vi "Find the extremal value using 2nd polynomial.vi"(5 "Y":dbl[](array[numeric]), 6 "X":dbl[](array[numeric])) -> (0 "Best Polynomial Fit":dbl[](array[numeric]), 1 "Polynomial Coefficients":dbl[](array[numeric]), 2 "Xm":dbl)   [LabVIEW 2014]
uses:
  <vilib>/Analysis/6fits.llb/General Linear Fit Algorithm.ctl
  <vilib>/Analysis/NI_AALPro.lvlib
panel:
  out "XY Graph":cluster{"X":dbl[], "Y":dbl[]}[](graph)
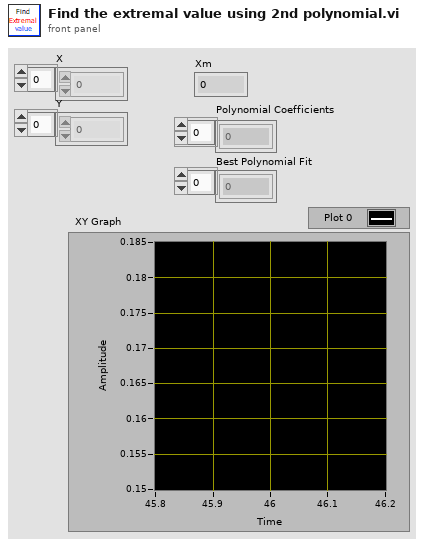
[diagram p1: front panel]
types:
  T1 = typedef "NI_AALPro.lvlib/General Linear Fit Algorithm.ctl" = u16
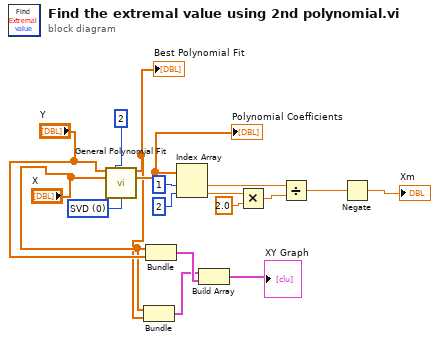
[diagram p0: block diagram]
diagram:
  w7 = T1 0 items=["SVD", "Givens", "Givens2", "Householder", "LU Decomposition", "Cholesky", "SVD for Rank Deficient H"] ("algorithm")
  n1 = call <vilib>:"General Polynomial Fit.vi"("Y"="Y", "polynomial order"=2, "X"="X", "algorithm"=w7) -> ("Best Polynomial Fit"=w4:dbl[], "Polynomial Coefficients"=w9:dbl[])  [unwired: 8 in, 2 out]
  "Best Polynomial Fit" <- w4
  "Polynomial Coefficients" <- w9
  n2 = Bundle("X"="X", "Best Polynomial Fit"=w4) -> (w2:cluster{"X":dbl[], "Best Polynomial Fit":dbl[]})  [unwired: 1 in]
  n3 = Bundle("X"="X", "Y"="Y") -> (w3:cluster{"X":dbl[], "Y":dbl[]})  [unwired: 1 in]
  n4 = Index Array(array=w9, index #1=1 ("index"), index #2=2 ("index")) -> (element #1=w14:dbl, element #2=w12:dbl)
  n5 = Build Array(w2, w3) -> (→"XY Graph":cluster{"X":dbl[], "Y":dbl[]}[])
  n6 = Multiply(x=w12, y=2.0) -> (x*y=w15:dbl)
  n7 = Divide(x=w14, y=w15) -> (x/y=w16:dbl)
  n8 = Negate(x=w16) -> (-x=→"Xm":dbl)
